vi "Get Boolean Notifier Ref.vi"(8 "error in (no error)":errorcluster, 9 "element data type":bool, 10 "Tag Name":string, 11 "Current Value Table in":refnum<class "Current Value Table.lvclass">) -> (0 "error out":errorcluster, 2 "notifier out":refnum<notifier>, 3 "Current Value Table out":refnum<class "Current Value Table.lvclass">)   [LabVIEW 2024, in "Current Value Table.lvlib" / "Current Value Table.lvclass"]
uses:
  Current Value Table.lvclass
  CVT_Boolean/CVT_Boolean.lvclass
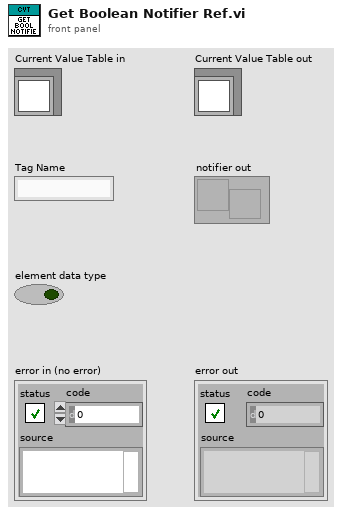
[diagram p1: front panel]
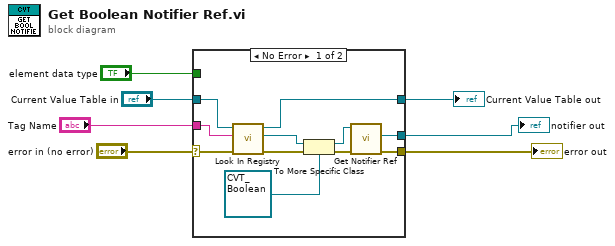
[diagram p0: block diagram]
diagram:
  n1 = case shown="No Error" "error in (no error)" {
    selector: "error in (no error)" -> [w12 w20]
    tunnel: [w14 w20] -> w6
    tunnel: [w8 w19] -> w4
    tunnel: "Current Value Table in" -> [w9 w19]
    tunnel: "Tag Name" -> [w13 _]
    tunnel: [w16 _] -> w2
    tunnel: "element data type" -> [_ _]
    frame No Error {
      n2 = call-dynamic "Look In Registry.vi"("error in (no error)"=w12, "Tag Name"=w13, "Current Value Table in"=w9) -> ("error out"=w11:errorcluster, "CVT_Item out"=w10:refnum<class "iCVT_Item.lvclass">, "Current Value Table out"=w8:refnum<class "Current Value Table.lvclass">)  [unwired: 5 in, 1 out]
      n3 = To More Specific Class(target class=refnum<class "CVT_Boolean.lvclass"> refnum ("CVT_Boolean in"), reference=w10, error in=w11) -> (specific class reference=w17:refnum<class "CVT_Boolean.lvclass">, error out=w15:errorcluster)
      n4 = call-dynamic "Get Notifier Ref.vi"("error in (no error)"=w15, "CVT_Boolean in"=w17) -> ("error out"=w14:errorcluster, "notifier out"=w16:refnum<notifier>)  [unwired: 7 in, 1 out]
    }
    frame Error {
    }
  }
  "error out" <- w6
  "Current Value Table out" <- w4
  "notifier out" <- w2
